vi "Call_Video_Still_with_Averaging.vi"(1 "Quality":u32=750 max=1000, 2 "Resolution":T1=1 items=["Low", "Med.", "High", "Max."]) -> (0 "Error out":errorcluster)   [LabVIEW 2016]
uses:
  Camera Server/Camera enum/Camera resolution.ctl
  Anemometry Sub Vis/Globals/Meas_global.vi
  Anemometry Sub Vis/Globals/Extra_Commands_Global.vi
  Camera Server/Globals/CamServer global.vi
  Anemometry Sub Vis/Globals/Trav_pos_global.vi
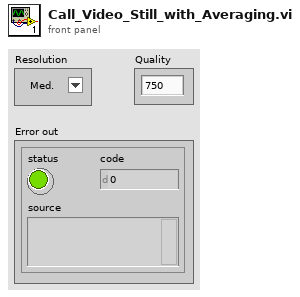
[diagram p1: front panel]
types:
  T1 = typedef "Camera resolution.ctl" = u8
  T2 = typedef "Camera enum.ctl" = string
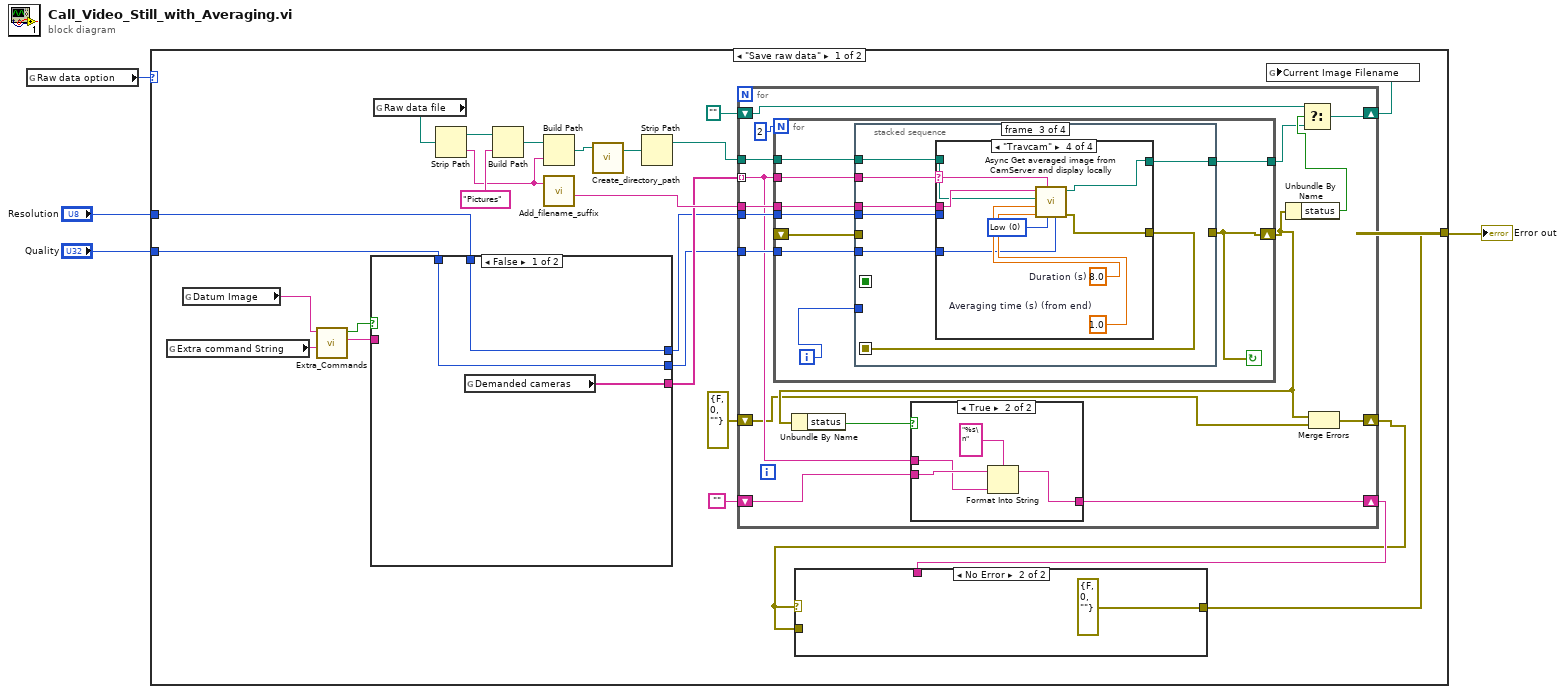
[diagram p0: block diagram]
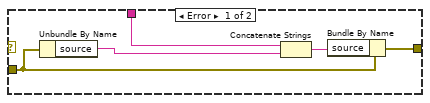
[diagram p2: hidden frame]
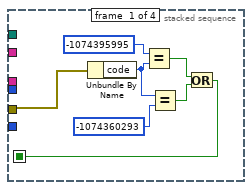
[diagram p4: hidden frame]
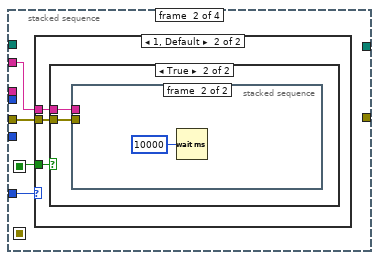
[diagram p5: hidden frame]
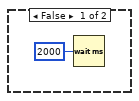
[diagram p7: hidden frame]
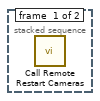
[diagram p8: hidden frame]
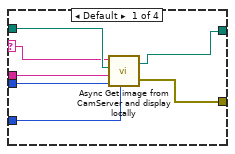
[diagram p9: hidden frame]
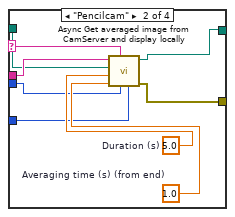
[diagram p10: hidden frame]
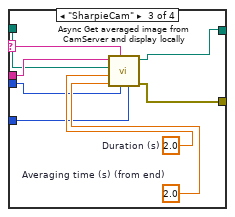
[diagram p11: hidden frame]
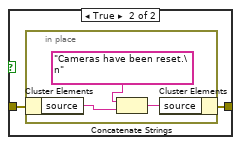
[diagram p14: hidden frame]
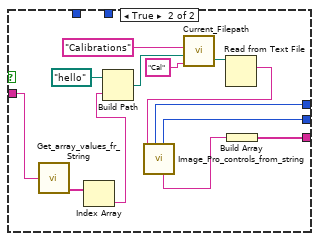
[diagram p15: hidden frame]
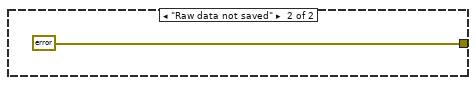
[diagram p16: hidden frame]
diagram:
  n1 = global read "Meas_global.vi" "Raw data option"() -> (w4:enum16{"Save raw data", "Raw data not saved"})
  n2 = case shown="\"Save raw data\"" w4 {
    tunnel: [w10 errorcluster {"status"=FALSE, "code"=0, "source"=""} ("Error out")] -> w3
    tunnel: "Resolution" -> [w13 _]
    tunnel: "Quality" -> [w12 _]
    frame "Save raw data" {
      n3 = global read "Meas_global.vi" "Extra command String"() -> (w16:string)
      n4 = global read "Extra_Commands_Global.vi" "Datum Image"() -> (w20:string)
      n5 = call "Extra_Commands.vi"("String to Search"=w16, "Command"=w20) -> ("String Value"=w17:string, "Command Found"=w19:bool)  [unwired: 2 in, 2 out]
      n6 = case shown="False" w19 {
        tunnel: [w140 w148] -> w18
        tunnel: w17 -> [_ w142]
        tunnel: [w138 w145] -> w15
        tunnel: [w139 w144] -> w14
        tunnel: w13 -> [w139 _]
        tunnel: w12 -> [w138 _]
        frame False {
          n7 = global read "CamServer global.vi" "Demanded cameras"() -> (w140:T2[])
        }
        frame True {
          n8 = call "Get_array_values_fr_String.vi"("String Value"=w142) -> ("String array"=w143:string[])  [unwired: 1 out]
          n9 = Index Array(array=w143) -> (element=w141:string)  [unwired: 1 in]
          n10 = Build Path(base path=path "hello", name or relative path=w141) -> (appended path=w149:path)
          n11 = call "Current_Filepath.vi"("Short_Name"="Cal" ("Data Type"), "Filename in"=w149, "Data Type"="Calibrations") -> ("Filename Out"=w153:path)  [unwired: 1 in, 1 out]
          n12 = Read from Text File(file (use dialog)=w153) -> (text=w147:string)  [unwired: 3 in, 3 out]
          n13 = call "Image_Pro_controls_from_string.vi"("Setup String"=w147) -> ("Camera"=w146:string, "Quality"=w145:u32, "Resolution"=w144:T1)  [unwired: 4 in, 4 out]
          n14 = Build Array(w146) -> (w148:string[])
        }
      }
      n15 = global read "Meas_global.vi" "Raw data file"() -> (w27:path)
      n16 = Strip Path(path=w27) -> (stripped path=w29:path, name=w23:string)
      n17 = Build Path(base path=w29, name or relative path="Pictures") -> (appended path=w26:path)
      n18 = Build Path(base path=w26, name or relative path=w23) -> (appended path=w25:path)
      n19 = call "Add_filename_suffix.vi"("Filename"=w23) -> ("Base name"=w22:string)  [unwired: 1 in, 3 out]
      n20 = call "Create_directory_path.vi"("Path name"=w25) -> ("Path name Out"=w24:path)  [unwired: 2 in, 1 out]
      n21 = Strip Path(path=w24) -> (stripped path=w21:path)  [unwired: 1 out]
      n22 = for {
        tunnel: w22 -> [w51]
        tunnel: w21 -> [w40]
        tunnel: w18 -> [w44] mode=indexing
        tunnel: w15 -> [w50]
        tunnel: w14 -> [w48]
        shift-right: [w46] -> w9
        shift-left: "" -> [w45]
        shift-right: [w41] -> w7
        shift-left: path "" -> [w42]
        shift-right: [w36] -> w5
        shift-left: errorcluster {"status"=FALSE, "code"=0, "source"=""} ("error IO") -> [w37]
        n23 = for {
          N: 2 -> [_]
          tunnel: w51 -> [w65]
          tunnel: w50 -> [w64]
          tunnel: w44 -> [w63]
          tunnel: w48 -> [w62]
          tunnel: w40 -> [w61]
          tunnel: [w60] -> w39
          shift-right: [w58] -> w38
          shift-left: _ -> [w57]
          i -> [w59]
          stop <- w58 continue-if-true
          n24 = stacked-sequence {
            seq-local: [w67 _ _ _] -> [_ w75 _ w125]
            seq-local: [_ _ w84 _] -> [_ _ _ w127]
            tunnel: w65 -> [_ _ w90 _]
            tunnel: w64 -> [_ _ w89 _]
            tunnel: w63 -> [_ w73 w88 _]
            tunnel: w62 -> [_ _ w87 _]
            tunnel: [_ _ _ w126] -> w58
            tunnel: w61 -> [_ _ w86 _]
            tunnel: [_ _ w85 _] -> w60
            tunnel: w59 -> [_ w76 _ _]
            tunnel: w57 -> [w72 w74 _ _]
            frame #0 {
              n25 = Unbundle By Name(w72) -> ("code"=w70:i32)
              n26 = Equal?(x=-1074395995, y=w70) -> (x = y?=w66:bool)
              n27 = Equal?(x=w70, y=-1074360293) -> (x = y?=w68:bool)
              n28 = Or(x=w66, y=w68) -> (x .or. y?=w67:bool)
            }
            frame #1 {
              n29 = case shown="1, Default" w76 {
                tunnel: w75 -> [_ w79]
                tunnel: w74 -> [_ w78]
                tunnel: w73 -> [_ w77]
                frame 0 {
                }
                frame 1, Default {
                  n30 = case shown="True" w79 {
                    tunnel: w78 -> [_ w82]
                    tunnel: w77 -> [_ w81]
                    frame False {
                      n31 = Wait (ms)(milliseconds to wait=u32 2000) -> ()  [unwired: 1 out]
                    }
                    frame True {
                      n32 = stacked-sequence {
                        tunnel: w82 -> [_ _]
                        tunnel: w81 -> [_ _]
                        frame #0 {
                          n33 = call "Call Remote Restart Cameras.vi"() -> ()  [unwired: 1 out]
                        }
                        frame #1 {
                          n34 = Wait (ms)(milliseconds to wait=u32 10000) -> ()  [unwired: 1 out]
                        }
                      }
                    }
                  }
                }
              }
            }
            frame #2 {
              n35 = case shown="\"Travcam\"" w88 {
                selector: w88 -> [w92 w99 w108 w118]
                tunnel: w90 -> [w97 w106 w115 w124]
                tunnel: w86 -> [w96 w105 w114 w123]
                tunnel: [w91 w98 w107 w117] -> w84
                tunnel: w89 -> [w95 w100 w109 w119]
                tunnel: [w94 w102 w111 w120] -> w85
                tunnel: w87 -> [w93 w101 w110 _]
                frame Default {
                  n36 = call "Async Get image from CamServer and display locally.vi"("Quality"=w95, "Resolution"=w93, "Image name"=w97, "Image directory path"=w96, "Camera"=w92) -> ("Error out"=w91:errorcluster, "Image file path"=w94:path)  [unwired: 1 in]
                }
                frame "Pencilcam" {
                  w103 = 1.0  # Averaging time (s) (from end)
                  w104 = 5.0  # Duration (s)
                  n37 = call "Async Get averaged image from CamServer and display locally.vi"("Quality"=w100, "Resolution"=w101, "Camera"=w99, "Averaging time (s) (from end)"=w103, "Duration (s)"=w104, "Image directory path"=w105, "Image name"=w106) -> ("Error out"=w98:errorcluster, "Image file path"=w102:path)  [unwired: 3 in]
                }
                frame "SharpieCam" {
                  w112 = 2.0  # Averaging time (s) (from end)
                  w113 = 2.0  # Duration (s)
                  n38 = call "Async Get averaged image from CamServer and display locally.vi"("Quality"=w109, "Resolution"=w110, "Camera"=w108, "Averaging time (s) (from end)"=w112, "Duration (s)"=w113, "Image directory path"=w114, "Image name"=w115) -> ("Error out"=w107:errorcluster, "Image file path"=w111:path)  [unwired: 3 in]
                }
                frame "Travcam" {
                  w116 = T1 0 items=["Low", "Med.", "High", "Max."] ("Resolution")
                  w121 = 1.0  # Averaging time (s) (from end)
                  w122 = 8.0  # Duration (s)
                  n39 = call "Async Get averaged image from CamServer and display locally.vi"("Quality"=w119, "Resolution"=w116, "Camera"=w118, "Averaging time (s) (from end)"=w121, "Duration (s)"=w122, "Image directory path"=w123, "Image name"=w124) -> ("Error out"=w117:errorcluster, "Image file path"=w120:path)  [unwired: 3 in]
                }
              }
            }
            frame #3 {
              n40 = case shown="No Error" w127 {
                tunnel: w127 -> [w128 w131]
                tunnel: [w128 w130] -> w126
                tunnel: w125 -> [_ w129]
                frame No Error {
                }
                frame Error {
                  n41 = case shown="False" w129 {
                    tunnel: w131 -> [w132 w134]
                    tunnel: [w132 w133] -> w130
                    frame False {
                    }
                    frame True {
                      n42 = in-place {
                        n43 = in-place-cluster #1(w134) -> ("source"=w137:string)
                        n44 = Concatenate Strings("Cameras have been reset.\n" ("format string"), w137) -> (w136:string)
                        n45 = in-place-cluster #1("source"=w136) -> (w133:errorcluster)
                      }
                    }
                  }
                }
              }
            }
          }
        }
        n46 = Unbundle By Name(w38) -> ("status"=w47:bool)
        n47 = case shown="True" w47 {
          tunnel: [w52 w54] -> w46
          tunnel: w45 -> [w52 w56]
          tunnel: w44 -> [_ w55]
          frame False {
          }
          frame True {
            n48 = Format Into String(format string="%s\n", initial string=w56, w55) -> (resulting string=w54:string)  [unwired: 1 in, 1 out]
          }
        }
        n49 = Unbundle By Name(w38) -> ("status"=w43:bool)
        n50 = Select(t=w42, s=w43, f=w39) -> (s? t:f=w41:path)
        n51 = Merge Errors(w38, w37) -> (w36:errorcluster)
      }
      n52 = case shown="No Error" w5 {
        tunnel: [w33 errorcluster {"status"=FALSE, "code"=0, "source"=""} ("Error out")] -> w10
        tunnel: w9 -> [w32 _]
        tunnel: w5 -> [w34 _]
        frame Error {
          n53 = Unbundle By Name(w34) -> ("source"=w31:string)
          n54 = Concatenate Strings(w32, w31) -> (w30:string)
          n55 = Bundle By Name(cluster=w34, "source"=w30) -> (w33:errorcluster)
        }
        frame No Error {
        }
      }
      n56 = global write "Trav_pos_global.vi" "Current Image Filename"(w7) -> ()
    }
    frame "Raw data not saved" {
    }
  }
  "Error out" <- w3
